vi "Send Process Calculation Results.vi"(7 "Message Priority (Normal)":T4=enum."Normal", 8 "error in (no error)":errorcluster, 10 "GPU Calculation Results":T1 {"Zoom Parameters"."fwidth:" format="%#_6p"; "Zoom Parameters"."f0:" format="%#_6p"}, 11 "Message Enqueuer":refnum<class "Message Enqueuer.lvclass">) -> (0 "error out":errorcluster, 3 "Message Enqueuer out":refnum<class "Message Enqueuer.lvclass">)   [LabVIEW 2020, in "GPU FFT Calculator.lvlib" / "Process Calculation Results Msg.lvclass"]
doc: "This VI sends the message to an actor."
uses:
  Process Calculation Results Msg.lvclass
  <vilib>/ActorFramework/Message Enqueuer/Message Enqueuer.lvclass
  <vilib>/ActorFramework/Message Enqueuer/Message Priority.ctl
  GPU FFT Calculator/GPU Calculation Message.ctl
  <vilib>/Natan Biesmans/G2CPU GPU and CPU HPC Toolkit/G2CPU Libraries/Async IO/DMA Manager/DMA Manager.lvclass
  <vilib>/Natan Biesmans/G2CPU GPU and CPU HPC Toolkit/G2CPU Libraries/Arrays/1DArray/s16/1D Array s16.lvclass
  <vilib>/Natan Biesmans/G2CPU GPU and CPU HPC Toolkit/G2CPU Libraries/Arrays/1DArray/f32/1D Array f32.lvclass
  chart zoom.ctl
  GPU FFT Calculator/GPU Metrics.ctl
  C:/Program Files/National Instruments/LabVIEW 2026/vi.lib/ActorFramework/Message/Message.lvclass
  Process Calculation Results Msg.lvclass/Process Calculation Results Msg.ctl
  <vilib>/ActorFramework/Message Enqueuer/Message Enqueuer.lvclass/Message Enqueuer.ctl
  <vilib>/ActorFramework/Message Priority Queue/Priority Enqueue.vi
  Simple UI/Simple UI/Simple UI.lvclass
  GPU FFT Calculator/GPU FFT Calculator.lvclass
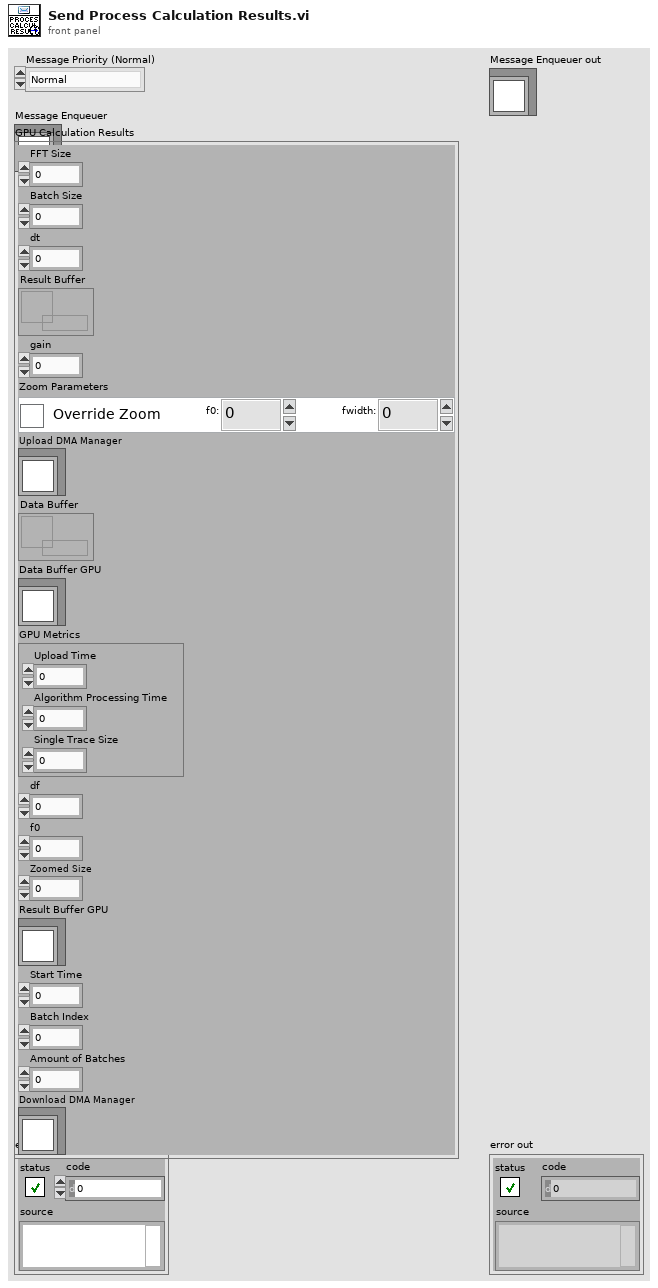
[diagram p1: front panel]
types:
  T1 = typedef "GPU FFT Calculator.lvlib/GPU FFT Calculator.lvclass/GPU Calculation Message.ctl" = cluster{"FFT Size":u64, "Batch Size":u64, "dt":dbl, "Result Buffer":refnum<data-value>, "gain":dbl, "Zoom Parameters":T2, "Upload DMA Manager":refnum<class "DMA Manager.lvclass">, "Data Buffer":refnum<data-value>, "Data Buffer GPU":refnum<class "1D Array s16.lvclass">, "GPU Metrics":T3, "df":dbl, "f0":dbl, "Zoomed Size":u64, "Result Buffer GPU":refnum<class "1D Array f32.lvclass">, "Start Time":dbl, "Batch Index":i32, "Amount of Batches":i32, "Download DMA Manager":refnum<class "DMA Manager.lvclass">}
  T2 = typedef "Simple UI.lvlib/Simple UI.lvclass/chart zoom.ctl" = cluster{"Override":bool, "f0: ":dbl, "fwidth: ":dbl}
  T3 = typedef "GPU FFT Calculator.lvlib/GPU FFT Calculator.lvclass/GPU Metrics.ctl" = cluster{"Upload Time":dbl, "Algorithm Processing Time":dbl, "Single Trace Size":u64}
  T4 = typedef "Actor Framework.lvlib/Message Enqueuer.lvclass/Message Priority.ctl" = enum16{"Low", "Normal", "High"}
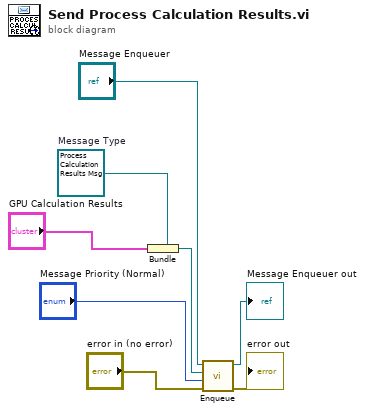
[diagram p0: block diagram]
diagram:
  w2 = refnum<class "Process Calculation Results Msg.lvclass"> refnum  # Message Type
  n1 = Bundle(cluster=w2, "GPU Calculation Results") -> (w3:refnum<class "Process Calculation Results Msg.lvclass">)
  n2 = call <vilib>:"Enqueue.vi"("error in (no error)"="error in (no error)", "Message Priority (Normal)"="Message Priority (Normal)", "Message"=w3, "Message Enqueuer in"="Message Enqueuer") -> ("error out"=→"error out":errorcluster, "Message Enqueuer out"=→"Message Enqueuer out":refnum<class "Message Enqueuer.lvclass">)  [unwired: 6 in]
